vi "CANOpen_Main_Initialize.vi"(7 "Enable SYNC":bool, 8 "error in (no error)":errorcluster, 9 "SDO Asynch":T1 {"HW Dyn Read"."Resp Chan."."Chan Refs" format="%.0x"; "HW Dyn Read"."Req Chan."."Chan Refs" format="%.0x"; "HW Dyn Write"."Resp Chan."."Chan Refs" format="%.0x"; "HW Dyn Write"."Req Chan."."Chan Refs" format="%.0x"; "List SDO"."Resp Chan."."Chan Refs" format="%.0x"; "List SDO"."Req Chan."."Chan Refs" format="%.0x"}, 10 "Nodes":T7[](array[typedef]) {"NMT"."Node init static SDO state" items=["start remote node"=1, "enter pre-operational"=128]; "NMT"."Node run state" items=["start remote node"=1, "stop remote node"=2, "enter pre-operational"=128, "reset node"=129, "reset communication"=130]; "Dynamic SDOs"."Sub-Index (0)" format="%.0x"; "Dynamic SDOs"."Object Index" format="%.0x"; "Dynamic SDOs"."Block Data" format="%.0x"; "RPDOs"."PDO Channel" items=["PDO 1", "PDO 2", "PDO 3", "PDO 4"]; "RPDOs"."Parameters"."Bit Offset" max=8 step=1; "RPDOs"."Parameters"."Byte Offset" max=8 step=1; "TPDOs"."PDO Channel" items=["PDO 1", "PDO 2", "PDO 3", "PDO 4"]; "TPDOs"."Parameters"."Bit Offset" max=8 step=1; "TPDOs"."Parameters"."Byte Offset" max=8 step=1; "SDOs"."Sub-Index (0)" format="%.0x"; "SDOs"."Object Index" format="%.0x"; "SDOs"."Block Data" format="%.0x"}, 11 "interface object":refnum<k20>) -> (0 "error out":errorcluster, 1 "xPDO Refs":T4, 2 "SYNC object out":refnum<k20>, 3 "interface object out":refnum<k20>, 4 "Security Ref":T3, 5 "Node States":u16[](array[ring]) items=["unknown"=1, "bootup"=0, "stopped"=4, "operational"=5, "pre-operational"=127, "connection lost"=128])   [LabVIEW 2021, in "CANOpen Addon Engine.lvlib"]
uses:
  CANOpen Addon Engine.lvlib
  SubVIS/CANOpen_Node Message Settings.ctl
  Shared/CANOpen_PDO Settings.ctl
  Shared/CANOpen_PDO Parameter Settings.ctl
  Shared/CANOpen_PDO Data Type.ctl
  System Explorer/SubVIs/CANopen Byte Order.ctl
  Shared/CANOpen_SDO Settings.ctl
  SubVIS/CANOpen_NMT Settings.ctl
  CanOpen_NMT_Config.ctl
  CanOpen_NMT_Static detect.ctl
  CANOpen_xPDO Refs.ctl
  CanOpen_RPDO Refs.ctl
  CanOpen_TPDO Refs.ctl
  CANOpen_HB_NG_EM Refs.ctl
  SubVIS/CANOpen_VS SDOs Data Refs.ctl
  <vilib>/NI VeriStand/Custom Device API/Data Reference.ctl
  CanOpen_SDO Dynamic queue.ctl
  Shared/CANOpen_SDO queue W data.ctl
  Shared/CANOpen_SDO queue mode.ctl
  Shared/CANOpen_PDO Data Type in queue.ctl
  <vilib>/CANopenLib/CANOPEN.llb/CANopen NMT Write.vi
  CANOpen_Check_Node_State.vi
  <vilib>/CANopenLib/CANOPEN.llb/CANopen SYNC Create.vi
  <vilib>/CANopenLib/CANOPEN.llb/CANopen SYNC Start.vi
  <vilib>/CANopenLib/CANOPEN.llb/CANopen TPDO Start.vi
  <vilib>/CANopenLib/CANOPEN.llb/CANopen RPDO Start.vi
  Shared/CANOpen Addon Shared.lvlib
  <vilib>/NI VeriStand/Custom Device API/Custom Device API.lvlib
  System Explorer/CANOpen Addon System Explorer.lvlib
panel:
  # "LSB"
  # "MSB"
  # "LSB"
  # "MSB"
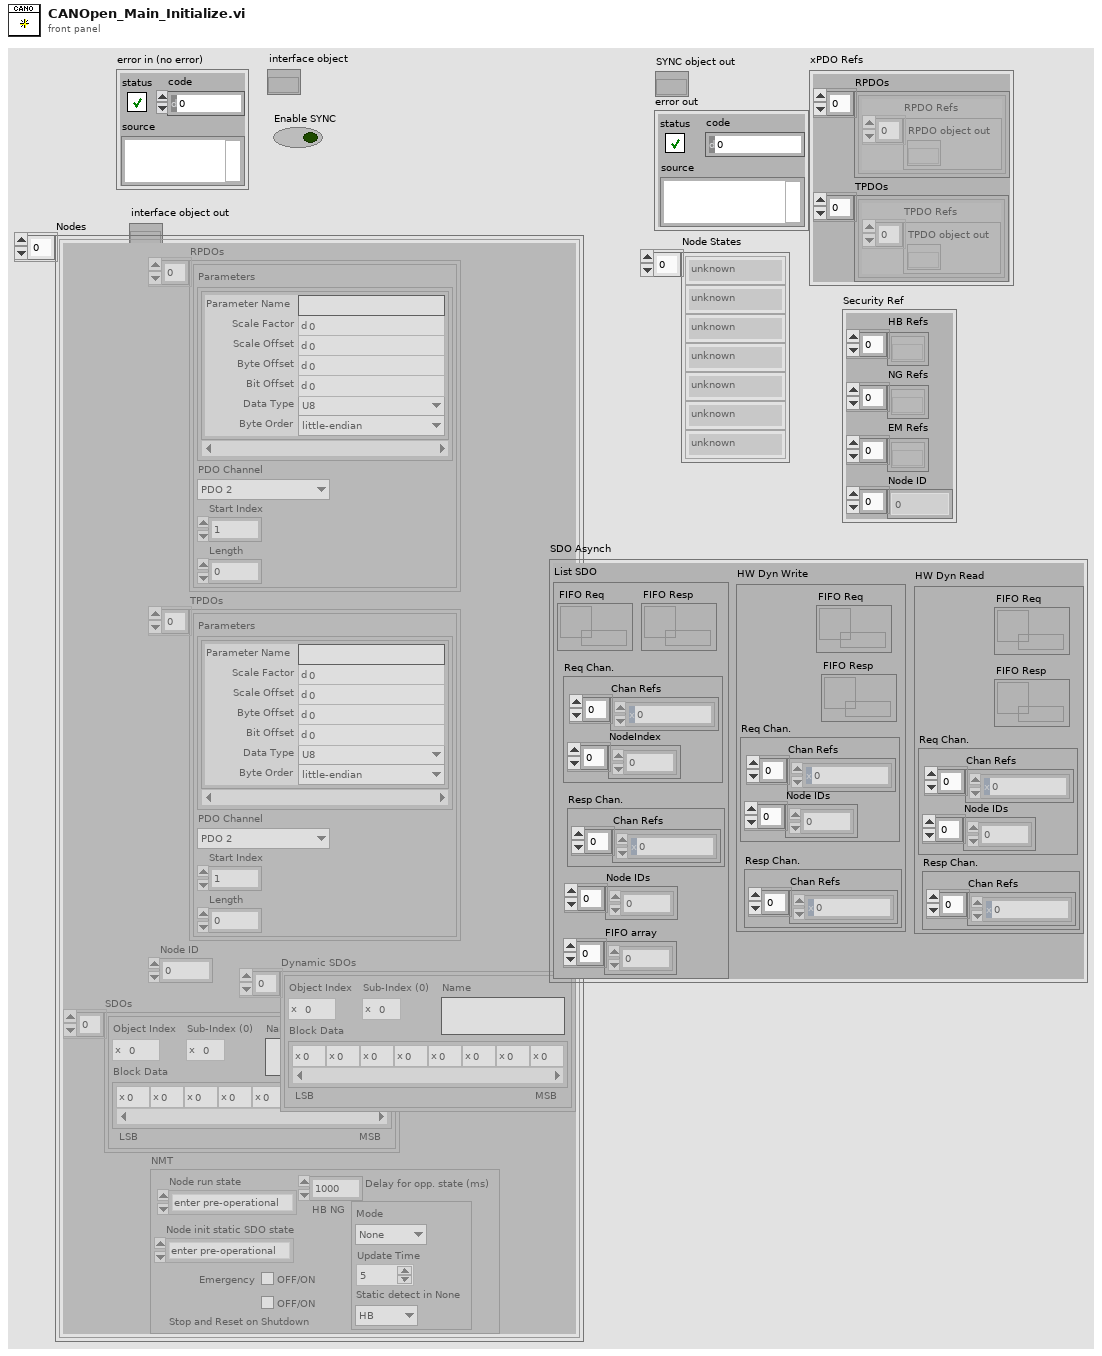
[diagram p1: front panel]
types:
  T1 = typedef "CANOpen Addon Engine.lvlib/CANOpen_VS SDOs Data Refs.ctl" = cluster{"List SDO":cluster{"FIFO Req":refnum<k33>, "Req Chan.":cluster{"Chan Refs":T2[], "NodeIndex":dbl[]}, "FIFO Resp":refnum<k33>, "Resp Chan.":cluster{"Chan Refs":T2[]}, "Node IDs":u8[], "FIFO array":dbl[]}, "HW Dyn Write":cluster{"FIFO Req":refnum<k33>, "FIFO Resp":refnum<k33>, "Req Chan.":cluster{"Chan Refs":T2[], "Node IDs":u8[]}, "Resp Chan.":cluster{"Chan Refs":T2[]}}, "HW Dyn Read":cluster{"FIFO Req":refnum<k33>, "FIFO Resp":refnum<k33>, "Req Chan.":cluster{"Chan Refs":T2[], "Node IDs":u8[]}, "Resp Chan.":cluster{"Chan Refs":T2[]}}}
  T2 = typedef "Custom Device API.lvlib/Data Reference.ctl" = i32
  T3 = typedef "CANOpen Addon Engine.lvlib/CANOpen_HB_NG_EM Refs.ctl" = cluster{"HB Refs":refnum<k20>[], "NG Refs":refnum<k20>[], "EM Refs":refnum<k20>[], "Node ID":u8[]}
  T4 = typedef "CANOpen Addon Engine.lvlib/CANOpen_xPDO Refs.ctl" = cluster{"RPDOs":T5[], "TPDOs":T6[]}
  T5 = typedef "CANOpen Addon Engine.lvlib/CanOpen_RPDO Refs.ctl" = cluster{"RPDO Refs":refnum<k20>[]}
  T6 = typedef "CANOpen Addon Engine.lvlib/CanOpen_TPDO Refs.ctl" = cluster{"TPDO Refs":refnum<k20>[]}
  T7 = typedef "CANOpen Addon Engine.lvlib/CANOpen_Node Message Settings.ctl" = cluster{"RPDOs":T8[], "TPDOs":T8[], "Node ID":u8, "SDOs":T12[], "Dynamic SDOs":T12[], "NMT":T13}
  T8 = typedef "CANOpen Addon Shared.lvlib/CANOpen_PDO Settings.ctl" = cluster{"Parameters":T9[], "PDO Channel":u8, "Start Index":u32, "Length":u32}
  T9 = typedef "CANOpen Addon Shared.lvlib/CANOpen_PDO Parameter Settings.ctl" = cluster{"Parameter Name":string, "Scale Factor":dbl, "Scale Offset":dbl, "Byte Offset":u8, "Bit Offset":u8, "Data Type":T10, "Byte Order":T11}
  T10 = typedef "CANOpen Addon Shared.lvlib/CANOpen_PDO Data Type.ctl" = enum16{"U8", "U16", "U32", "I8", "I16", "I32", "Single", "Double", "Boolean"}
  T11 = typedef "CANOpen Addon System Explorer.lvlib/CANopen Byte Order.ctl" = enum16{"big-endian network order", "little-endian"}
  T12 = typedef "CANOpen Addon Shared.lvlib/CANOpen_SDO Settings.ctl" = cluster{"Object Index":u16, "Sub-Index (0)":u8, "Block Data":u8[], "Name":string}
  T13 = typedef "CANOpen Addon Engine.lvlib/CANOpen_NMT Settings.ctl" = cluster{"Node run state":u16, "Emergency":bool, "HB NG":T14, "Delay for opp. state (ms)":dbl, "Node init static SDO state":u16, "Stop and Reset on Shutdown":bool}
  T14 = typedef "CANOpen Addon Engine.lvlib/CanOpen_NMT_Config.ctl" = cluster{"Mode":T15, "Update Time":u16, "Static detect in None":T15}
  T15 = typedef "CANOpen Addon Engine.lvlib/CanOpen_NMT_Static detect.ctl" = enum16{"None", "HB", "NG"}
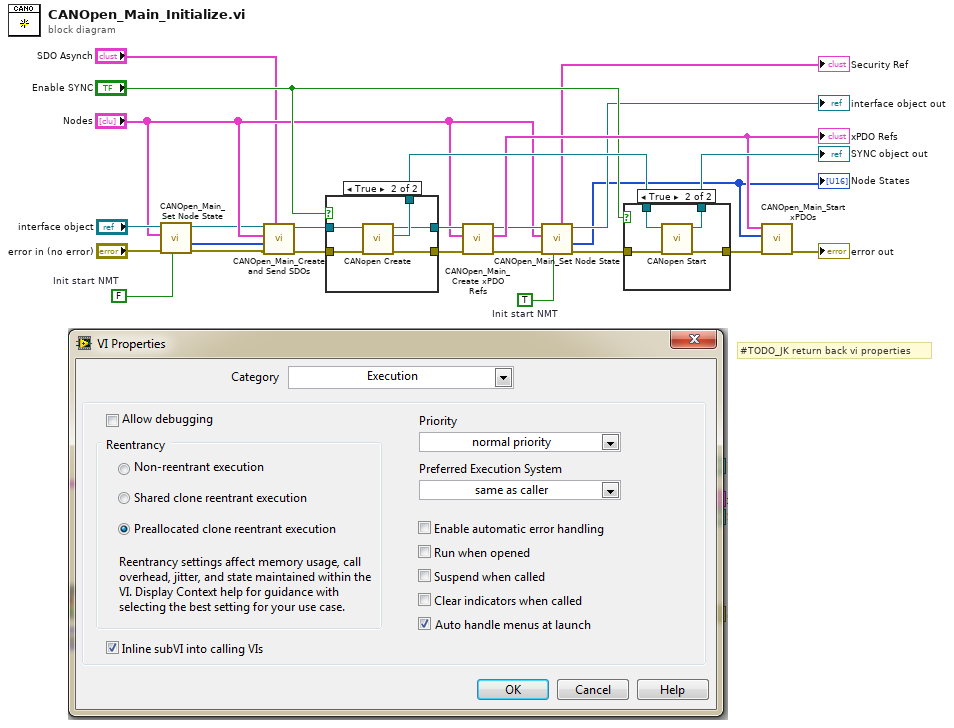
[diagram p0: block diagram]
diagram:
  w3 = FALSE  # Init start NMT
  w4 = TRUE  # Init start NMT
  # "#TODO_JK return back vi properties"
  n1 = call "CANOpen_Main_Set Node State.vi"("Start NMT"=w3, "error in (no error)"="error in (no error)", "Nodes"="Nodes", "interface object"="interface object") -> ("error out"=w7:errorcluster, "States"=w15:u16[], "interface object out"=w6:refnum<k20>)  [unwired: 4 in, 1 out]
  n2 = call "CANOpen_Main_Create and Send SDOs.vi"("SDO Asynch"="SDO Asynch", "error in (no error)"=w7, "Node States"=w15, "Nodes"="Nodes", "interface object"=w6) -> ("error out"=w17:errorcluster, "interface object out"=w18:refnum<k20>)  [unwired: 5 in]
  n3 = case shown="True" "Enable SYNC" {
    tunnel: [_ w32] -> w24
    tunnel: [w27 w31] -> w21
    tunnel: [w26 w30] -> w20
    tunnel: w18 -> [w27 w29]
    tunnel: w17 -> [w26 w28]
    frame False {
    }
    frame True {
      n4 = call-poly <vilib>:"CANopen Create.vi"("error in (no error)"=w28, "interface object in"=w29) -> ("error out"=w30:errorcluster, "SYNC object out"=w32:refnum<k20>, "interface object out"=w31:refnum<k20>)  [unwired: 7 in]
    }
  }
  n5 = call "CANOpen_Main_Create xPDO Refs.vi"("error in (no error)"=w20, "Nodes"="Nodes", "interface object"=w21) -> ("error out"=w12:errorcluster, "xPDO Refs"=w19:T4, "interface object out"=w11:refnum<k20>)  [unwired: 6 in]
  "xPDO Refs" <- w19
  n6 = call "CANOpen_Main_Set Node State.vi"("Start NMT"=w4, "error in (no error)"=w12, "Nodes"="Nodes", "interface object"=w11) -> ("error out"=w10:errorcluster, "States"=w5:u16[], "interface object out"=→"interface object out":refnum<k20>, "Security Ref"=→"Security Ref":T3)  [unwired: 4 in]
  "Node States" <- w5
  n7 = case shown="True" "Enable SYNC" {
    tunnel: [w33 w38] -> w25
    tunnel: w24 -> [w33 w37]
    tunnel: [w34 w36] -> w23
    tunnel: w10 -> [w34 w35]
    frame False {
    }
    frame True {
      n8 = call-poly <vilib>:"CANopen Start.vi"("error in (no error)"=w35, "SYNC object in"=w37) -> ("error out"=w36:errorcluster, "SYNC object out"=w38:refnum<k20>)  [unwired: 8 in]
    }
  }
  "SYNC object out" <- w25
  n9 = call "CANOpen_Main_Start xPDOs.vi"("error in (no error)"=w23, "States"=w5, "xPDO Refs"=w19) -> ("error out"=→"error out":errorcluster)  [unwired: 8 in]
